vi "Read_header.vi"(8 "error in (no error)":errorcluster, 11 "HIS in":refnum<class "HIS.lvclass">) -> (0 "error out":errorcluster, 1 "TimeDelays,pixels":i32, 2 "Wavelength, pixels":i32, 3 "HIS out":refnum<class "HIS.lvclass">, 4 "ScalingYScalingFile":i64=1060864, 5 "ScalingXScalingFile":i64=1058816, 6 "size bytes per number":i8, 7 "#Images":i32, 9 "comments":u16)   [LabVIEW 2019, in "HIS.lvclass"]
uses:
  HIS.lvclass
  C:/Users/elysium/Documents/dev/TRANCON/Classes/DATA/DATA.lvclass
  DATA.lvclass/DATA.ctl
  DATA.lvclass
panel:
  out "Timescale":i32
  out "Wavelength":dbl
  out "ScalingYScale":dbl
  out "Time delay unit":string
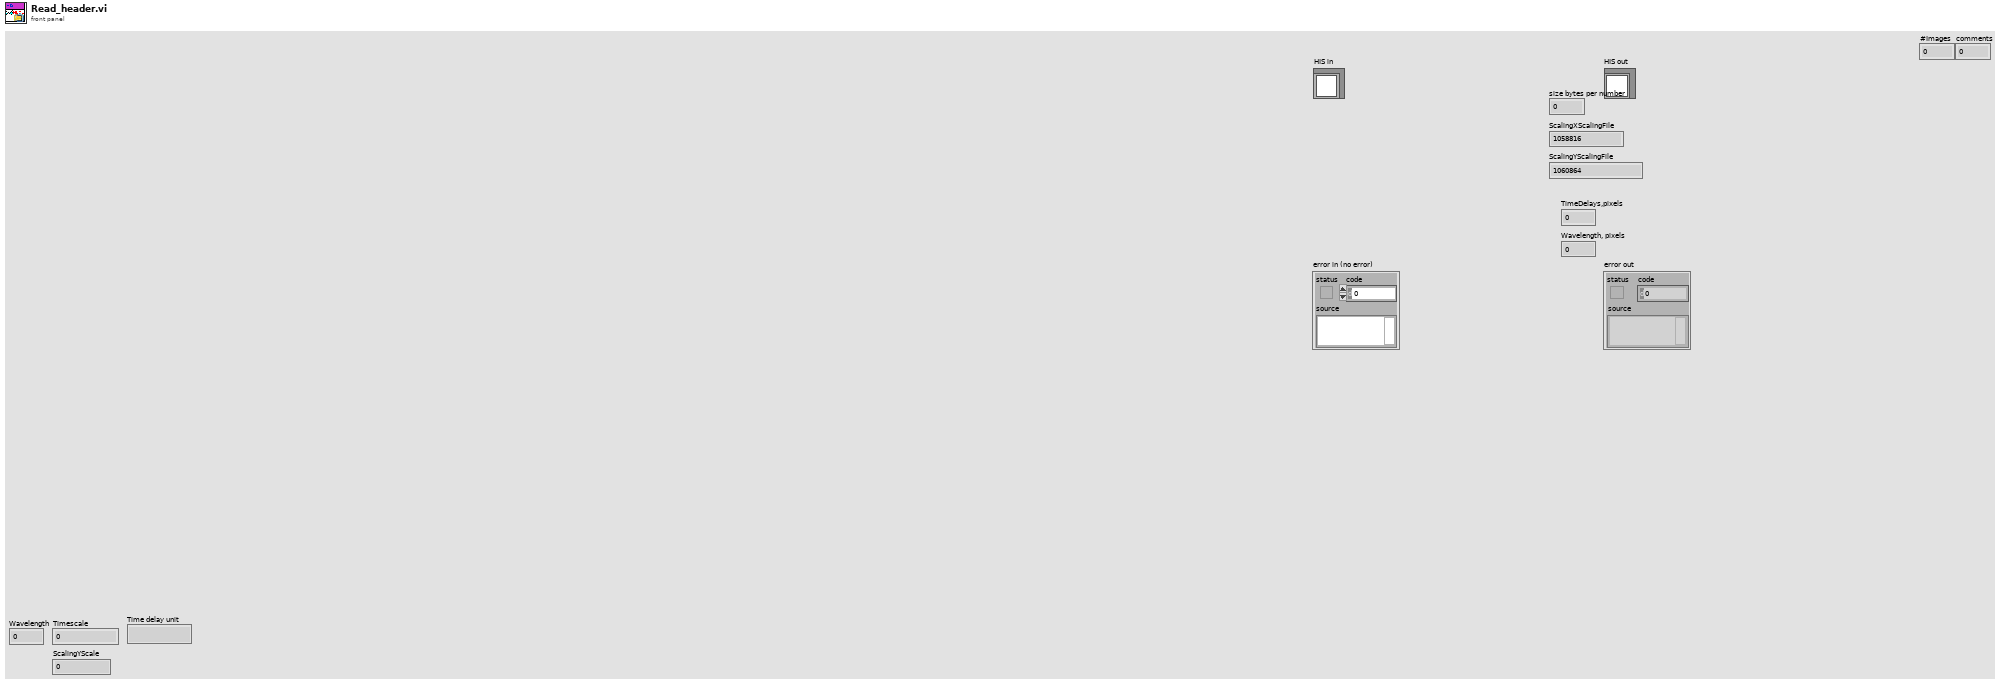
[diagram p1: front panel]
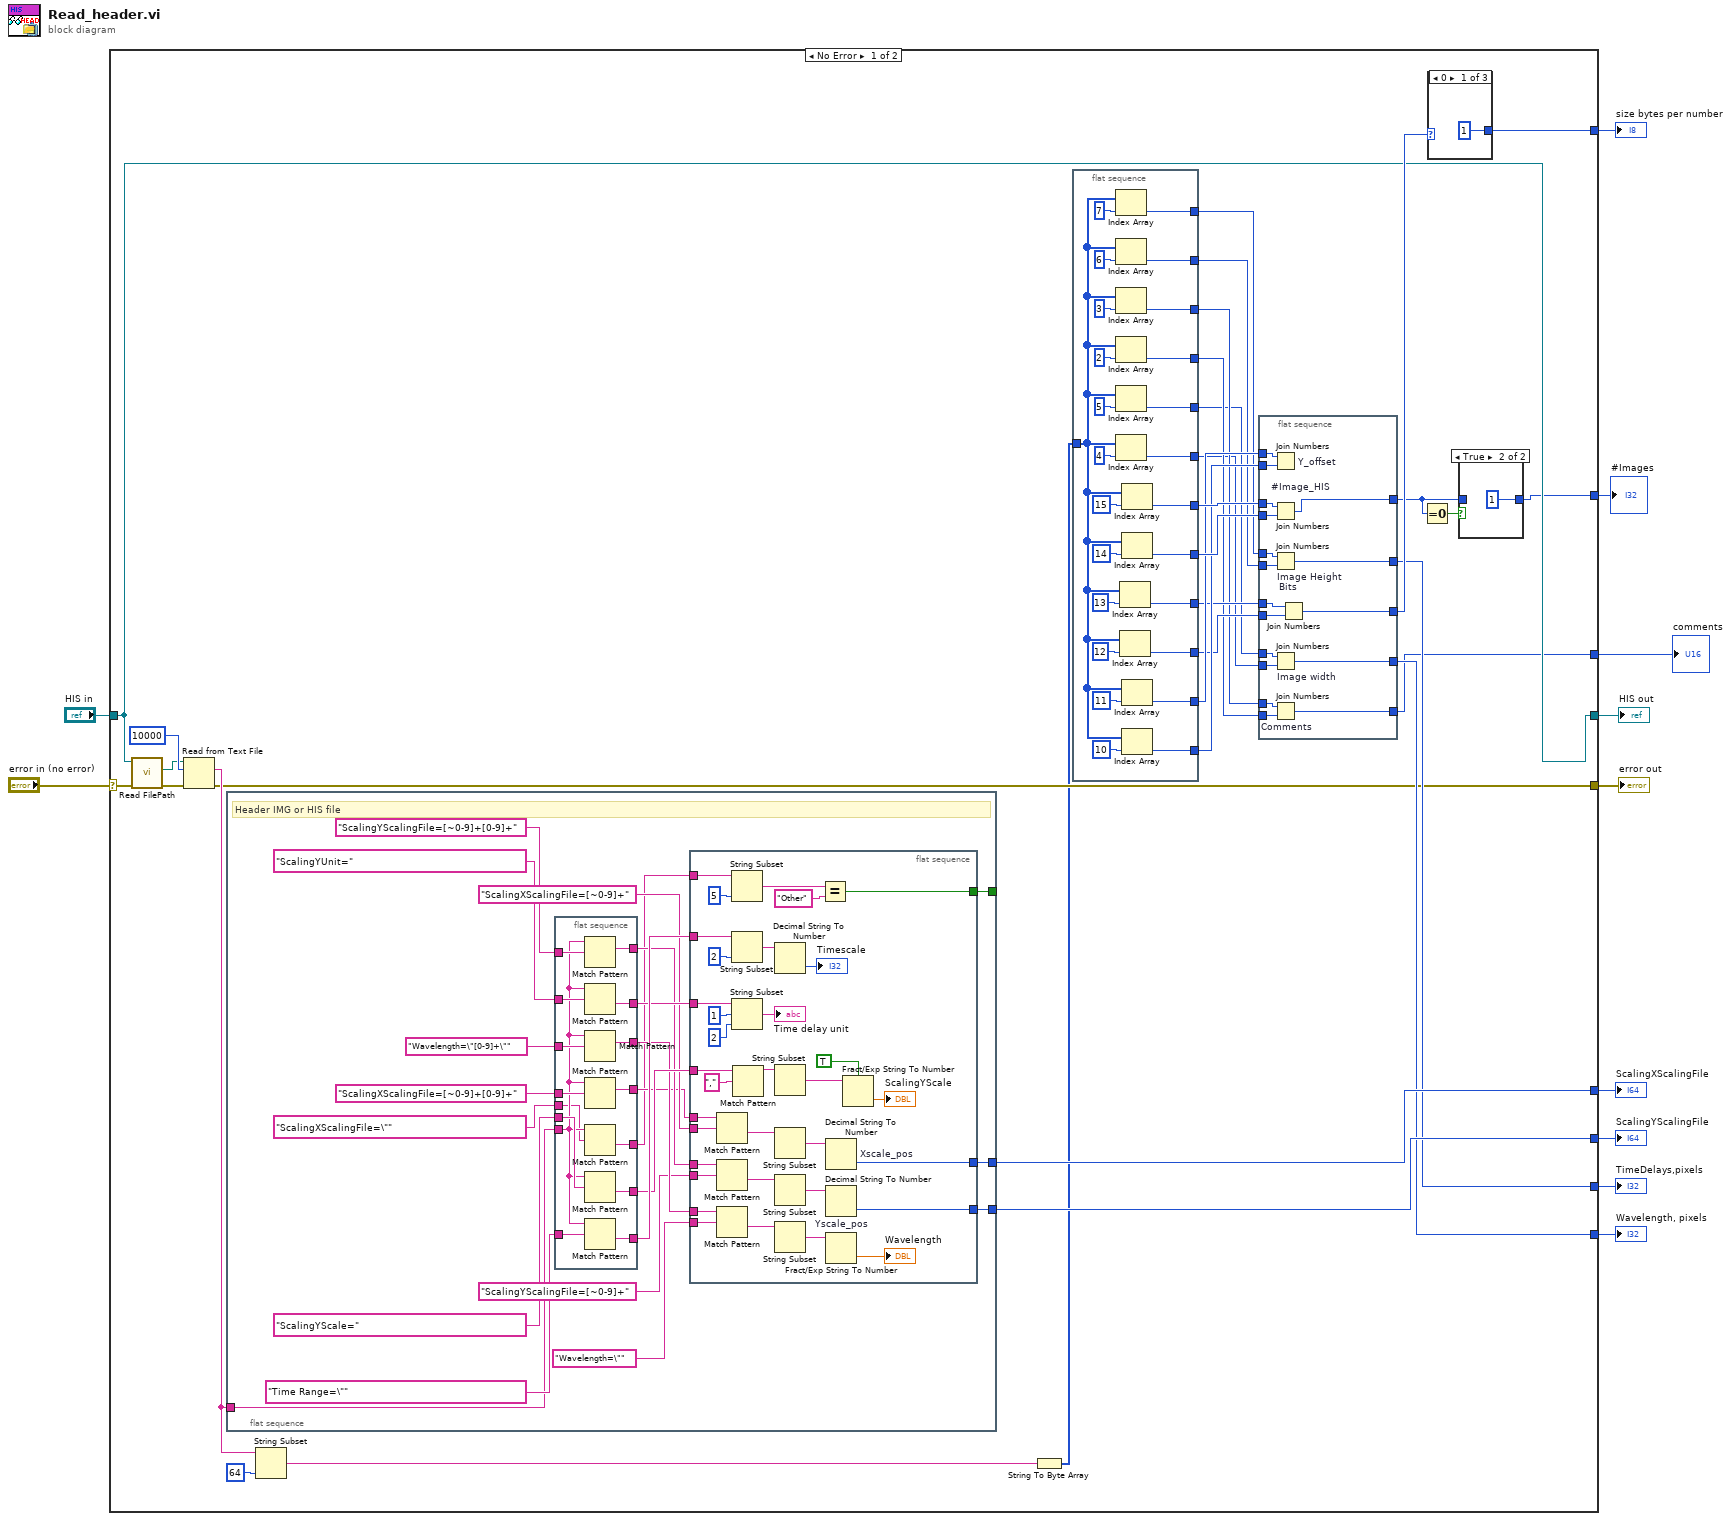
[diagram p0: block diagram]
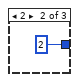
[diagram p3: hidden frame]
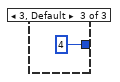
[diagram p4: hidden frame]
diagram:
  n1 = case shown="No Error" "error in (no error)" {
    selector: "error in (no error)" -> [w20 w162]
    tunnel: [w15 w162] -> w10
    tunnel: [w16 w161] -> w8
    tunnel: "HIS in" -> [w16 w161]
    tunnel: [w25 _] -> w7
    tunnel: [w24 _] -> w6
    tunnel: [w23 _] -> w5
    tunnel: [w22 _] -> w4
    tunnel: [w21 _] -> w3
    tunnel: [w14 _] -> w2
    tunnel: [w13 _] -> w1
    frame No Error {
      n2 = call "Read FilePath.vi"("error in (no error)"=w20, "DATA in"=w16) -> ("error out"=w27:errorcluster, "FilePath"=w26:path)  [unwired: 7 in, 1 out]
      n3 = Read from Text File(file (use dialog)=w26, count=10000, error in=w27) -> (text=w19:string, error out=w15:errorcluster)  [unwired: 1 in, 2 out]
      n4 = flat-sequence {
        tunnel: [w105] -> _
        tunnel: [w104] -> w25
        tunnel: w19 -> [w91]
        tunnel: [w88] -> w24
        frame #0 {
          # "Header IMG or HIS file"
          n5 = flat-sequence {
            tunnel: "Time Range=\"" -> [w157]
            tunnel: [w156] -> w107
            tunnel: "ScalingYScale=" -> [w155]
            tunnel: "ScalingYScalingFile=[~0-9]+[0-9]+" ("String 2") -> [w154]
            tunnel: [w153] -> w102
            tunnel: "ScalingYUnit=" -> [w152]
            tunnel: [w151] -> w100
            tunnel: "Wavelength=\"[0-9]+\"" -> [w150]
            tunnel: [w149] -> w98
            tunnel: [w148] -> w95
            tunnel: "ScalingXScalingFile=[~0-9]+[0-9]+" ("String 2") -> [w147]
            tunnel: [w146] -> w92
            tunnel: w91 -> [w145]
            tunnel: [w144] -> w90
            tunnel: "ScalingXScalingFile=\"" -> [w143]
            frame #0 {
              n6 = Match Pattern(string=w145, regular expression=w154) -> (match substring=w148:string)  [unwired: 1 in, 3 out]
              n7 = Match Pattern(string=w145, regular expression=w152) -> (after substring=w151:string)  [unwired: 1 in, 3 out]
              n8 = Match Pattern(string=w145, regular expression=w150) -> (match substring=w149:string)  [unwired: 1 in, 3 out]
              n9 = Match Pattern(string=w145, regular expression=w147) -> (match substring=w146:string)  [unwired: 1 in, 3 out]
              n10 = Match Pattern(string=w145, regular expression=w143) -> (after substring=w144:string)  [unwired: 1 in, 3 out]
              n11 = Match Pattern(string=w145, regular expression=w155) -> (after substring=w153:string)  [unwired: 1 in, 3 out]
              n12 = Match Pattern(string=w145, regular expression=w157) -> (after substring=w156:string)  [unwired: 1 in, 3 out]
            }
          }
          n13 = flat-sequence {
            tunnel: w107 -> [w142]
            tunnel: [w135] -> w105
            tunnel: [w129] -> w104
            tunnel: w102 -> [w128]
            tunnel: w100 -> [w125]
            tunnel: w98 -> [w121]
            tunnel: "Wavelength=\"" ("String") -> [w120]
            tunnel: "ScalingYScalingFile=[~0-9]+" ("regular expression") -> [w118]
            tunnel: w95 -> [w117]
            tunnel: "ScalingXScalingFile=[~0-9]+" ("regular expression") -> [w115]
            tunnel: w92 -> [w114]
            tunnel: w90 -> [w113]
            tunnel: [w109] -> w88
            frame #0 {
              n14 = Match Pattern(string=w114, regular expression=w115) -> (after substring=w116:string)  [unwired: 1 in, 3 out]
              n15 = Match Pattern(string=w117, regular expression=w118) -> (after substring=w111:string)  [unwired: 1 in, 3 out]
              n16 = Match Pattern(string=w121, regular expression=w120) -> (after substring=w119:string)  [unwired: 1 in, 3 out]
              n17 = String Subset(string=w113, length (rest)=5 ("length (rest)")) -> (substring=w134:string)  [unwired: 1 in]
              n18 = String Subset(string=w142, length (rest)=2 ("length (rest)")) -> (substring=w140:string)  [unwired: 1 in]
              n19 = String Subset(string=w125, offset (0)=1, length (rest)=2 ("length (rest)")) -> (substring=→"Time delay unit":string)
              n20 = Match Pattern(string=w128, regular expression=",") -> (before substring=w126:string)  [unwired: 1 in, 3 out]
              n21 = Decimal String To Number(string=w140) -> (number=→"Timescale":i32)  [unwired: 2 in, 1 out]
              n22 = String Subset(string=w126) -> (substring=w137:string)  [unwired: 2 in]
              n23 = String Subset(string=w116) -> (substring=w130:string)  [unwired: 2 in]
              n24 = String Subset(string=w111) -> (substring=w110:string)  [unwired: 2 in]
              n25 = String Subset(string=w119) -> (substring=w138:string)  [unwired: 2 in]
              n26 = Equal?(x=w134, y="Other") -> (x = y?=w135:bool)
              n27 = Decimal String To Number "Xscale_pos"(string=w130) -> (number=w129:i32)  [unwired: 2 in, 1 out]
              n28 = Decimal String To Number "Yscale_pos"(string=w110) -> (number=w109:i32)  [unwired: 2 in, 1 out]
              n29 = Fract/Exp String To Number(string=w138) -> (number=→"Wavelength":dbl)  [unwired: 3 in, 1 out]
              n30 = Fract/Exp String To Number(use system decimal point (T)=TRUE, string=w137) -> (number=→"ScalingYScale":dbl)  [unwired: 2 in, 1 out]
            }
          }
        }
      }
      n31 = String Subset(string=w19, length (rest)=64 ("length (rest)")) -> (substring=w17:string)  [unwired: 1 in]
      n32 = String To Byte Array(string=w17) -> (unsigned byte array=w12:u8[])
      n33 = flat-sequence {
        tunnel: [w87] -> w28
        tunnel: [w86] -> w29
        tunnel: [w85] -> w30
        tunnel: [w84] -> w31
        tunnel: [w83] -> w32
        tunnel: [w82] -> w33
        tunnel: [w79] -> w34
        tunnel: [w78] -> w35
        tunnel: [w71] -> w36
        tunnel: [w70] -> w37
        tunnel: [w65] -> w39
        tunnel: [w64] -> w40
        tunnel: w12 -> [w63]
        frame #0 {
          n34 = Index Array(array=w63, index=7 ("Index")) -> (element=w78:u8)
          n35 = Index Array(array=w63, index=6 ("Index")) -> (element=w79:u8)
          n36 = Index Array(array=w63, index=3 ("Index")) -> (element=w84:u8)
          n37 = Index Array(array=w63, index=2 ("Index")) -> (element=w85:u8)
          n38 = Index Array(array=w63, index=5 ("Index")) -> (element=w87:u8)
          n39 = Index Array(array=w63, index=4 ("Index")) -> (element=w86:u8)
          n40 = Index Array(array=w63, index=13 ("Index")) -> (element=w82:u8)
          n41 = Index Array(array=w63, index=12 ("Index")) -> (element=w83:u8)
          n42 = Index Array(array=w63, index=15) -> (element=w65:u8)
          n43 = Index Array(array=w63, index=14) -> (element=w64:u8)
          n44 = Index Array(array=w63, index=11) -> (element=w70:u8)
          n45 = Index Array(array=w63, index=10) -> (element=w71:u8)
        }
      }
      n46 = flat-sequence {
        tunnel: w28 -> [w62]
        tunnel: w29 -> [w61]
        tunnel: w30 -> [w60]
        tunnel: w31 -> [w59]
        tunnel: w32 -> [w58]
        tunnel: w33 -> [w57]
        tunnel: [w56] -> w13
        tunnel: w34 -> [w55]
        tunnel: w35 -> [w54]
        tunnel: w36 -> [w53]
        tunnel: w37 -> [w52]
        tunnel: w39 -> [w51]
        tunnel: w40 -> [w50]
        tunnel: [w49] -> w43
        tunnel: [w48] -> w23
        tunnel: [w47] -> w22
        tunnel: [w46] -> w42
        frame #0 {
          n47 = Join Numbers "Y_offset"(hi=w52, lo=w53) -> ()  [unwired: 1 out]
          n48 = Join Numbers "#Image_HIS"(hi=w51, lo=w50) -> ((hi.lo)=w46:u16)
          n49 = Join Numbers "Image Height"(hi=w54, lo=w55) -> ((hi.lo)=w47:u16)
          n50 = Join Numbers "Image width"(hi=w62, lo=w61) -> ((hi.lo)=w48:u16)
          n51 = Join Numbers "Comments"(hi=w59, lo=w60) -> ((hi.lo)=w56:u16)
          n52 = Join Numbers "Bits"(hi=w57, lo=w58) -> ((hi.lo)=w49:u16)
        }
      }
      n53 = Equal To 0?(x=w42) -> (x = 0?=w41:bool)
      n54 = case shown="0" w43 {
        tunnel: [i8 1 i8 2 i8 4] -> w21
        frame 0 {
        }
        frame 2 {
        }
        frame 3, Default {
        }
      }
      n55 = case shown="True" w41 {
        tunnel: [w44 1] -> w14
        tunnel: w42 -> [w44 _]
        frame False {
        }
        frame True {
        }
      }
    }
    frame Error {
    }
  }
  "error out" <- w10
  "HIS out" <- w8
  "ScalingYScalingFile" <- w6
  "ScalingXScalingFile" <- w7
  "Wavelength, pixels" <- w5
  "TimeDelays,pixels" <- w4
  "size bytes per number" <- w3
  "#Images" <- w2
  "comments" <- w1
